vi "RandomDouble.vi"(10 "Min":dbl, 11 "Max":dbl) -> (3 "Random":dbl)   [LabVIEW 2013]
doc: "Gives a random number between the two inputs, inclusive. \"Max\" can actually be smaller than \"Min,\" in this case, a random number [Max, Min] is given."
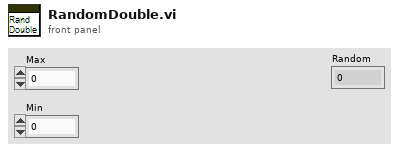
[diagram p1: front panel]
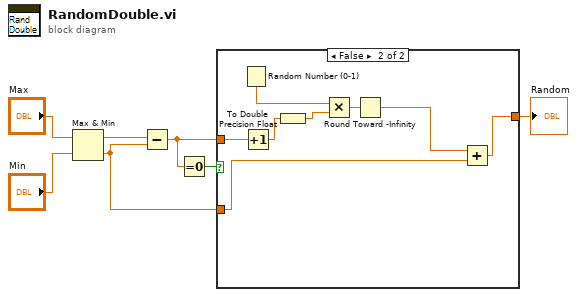
[diagram p0: block diagram]
diagram:
  n1 = Max & Min(x="Max", y="Min") -> (max(x,y)=w4:dbl, min(x,y)=w1:dbl)
  n2 = Subtract(x=w4, y=w1) -> (x-y=w3:dbl)
  n3 = Equal To 0?(x=w3) -> (x = 0?=w2:bool)
  n4 = case shown="False" w2 {
    tunnel: [w8 w15] -> w7
    tunnel: w3 -> [_ w11]
    tunnel: w1 -> [w8 w10]
    frame True {
    }
    frame False {
      n5 = Random Number (0-1)() -> (number: 0 to 1=w16:dbl)
      n6 = Increment(x=w11) -> (x+1=w14:dbl)
      n7 = To Double Precision Float(number=w14) -> (double precision float=w13:dbl)
      n8 = Multiply(x=w16, y=w13) -> (x*y=w12:dbl)
      n9 = Round Toward -Infinity(1:w12) -> (0:w9:dbl)
      n10 = Add(x=w9, y=w10) -> (x+y=w15:dbl)
    }
  }
  "Random" <- w7
